vi "Actuators Move Relative Channel.vi"(0 "Notifier Name":string, 2 "Wait to Finish":bool, 5 "Channel":i32, 7 "Step":dbl, 11 "Error In":errorcluster) -> (4 "Notifier Name Out":string, 6 "Channel Out":i32, 15 "Error Out":errorcluster)   [LabVIEW 2025]
uses:
  Actuators Controls/Actuators Note Type.ctl
  Actuators Controls/Actuators Actions.ctl
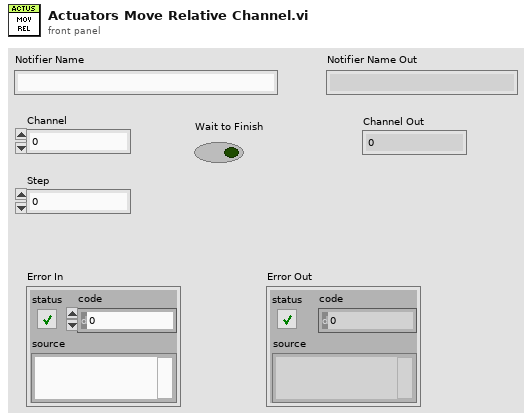
[diagram p1: front panel]
types:
  T1 = typedef "Actuators Note Type.ctl" = cluster{"Actions":T2, "Cmd Received ":bool, "Setpoint":dbl[], "Position":dbl[], "Channel":i32[], "Jog Step":dbl[], "Velocity":dbl[], "Acceleration":dbl[], "Status Bits":u32[], "Moving":bool[]}
  T2 = typedef "Actuators Actions.ctl" = enum16{"Nothing", "Get Position", "Get Acceleration", "Get Velocity", "Get Jog Step", "Set Acceleration", "Set Velocity", "Set Jog Step", "Move Absolute", "Move Relative", "Jog Forward", "Jog Reverse", "Set Moving", "Halt", "Quit"}
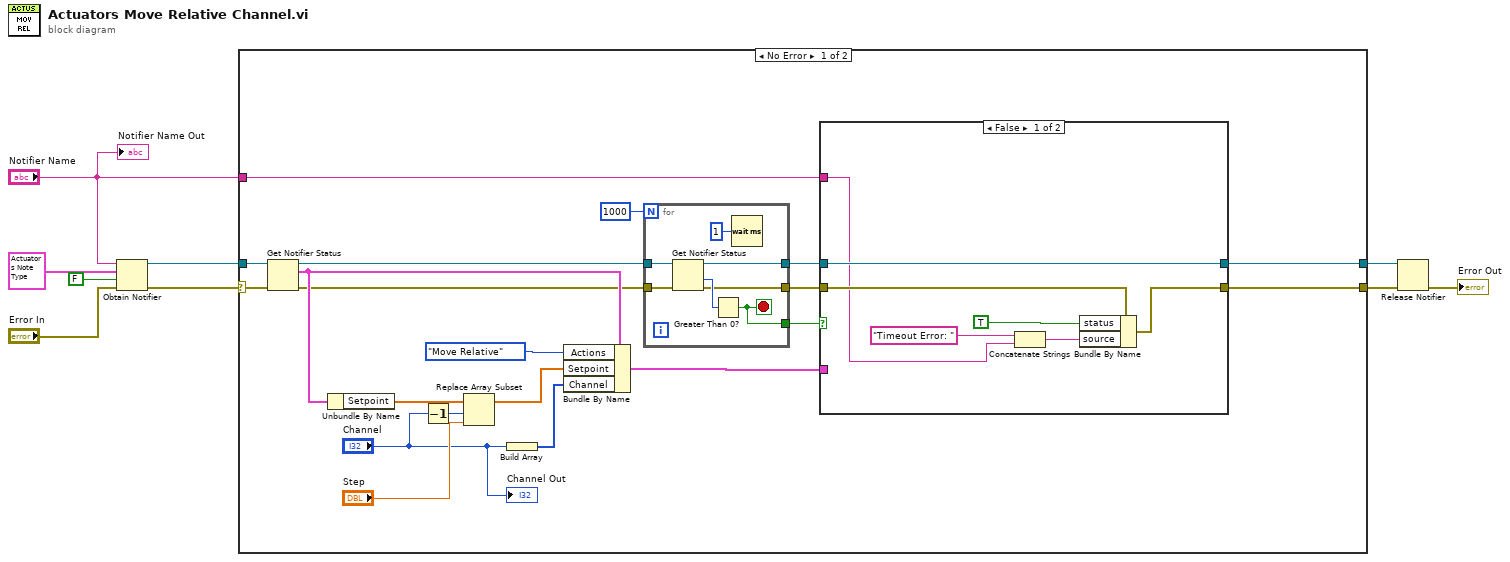
[diagram p0: block diagram]
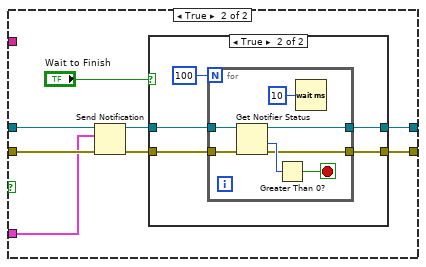
[diagram p2: hidden frame]
diagram:
  n1 = Obtain Notifier(name (unnamed)="Notifier Name", notification data type=T1 {"Actions"=enum."Nothing", "Cmd Received "=FALSE, "Setpoint"=[], "Position"=[], "Channel"=[], "Jog Step"=[], "Velocity"=[], "Acceleration"=[], "Status Bits"=[], "Moving"=[]} ("Actuators Note"), create if not found? (T)=FALSE, error in (no error)="Error In") -> (notifier out=w5:refnum<notifier>, error out=w8:errorcluster)  [unwired: 1 out]
  n2 = case shown="No Error" w8 {
    selector: w8 -> [w23 w66]
    tunnel: w5 -> [w24 w67]
    tunnel: "Notifier Name" -> [w14 _]
    tunnel: [w29 w67] -> w4
    tunnel: [w28 w66] -> w3
    frame No Error {
      n3 = Get Notifier Status(notifier=w24, error in (no error)=w23) -> (notifier out=w20:refnum<notifier>, current notification=w22:T1, error out=w19:errorcluster)  [unwired: 2 out]
      n4 = Unbundle By Name(w22) -> ("Setpoint"=w26:dbl[])
      n5 = Decrement(x="Channel") -> (x-1=w11:i32)
      n6 = Replace Array Subset(array=w26, new element="Step", index=w11) -> (w27:dbl[])
      n7 = Build Array("Channel") -> (w13:i32[])
      n8 = Bundle By Name(cluster=w22, "Actions"=Actuators_Actions."Move Relative", "Setpoint"=w27, "Channel"=w13) -> (w15:T1)
      n9 = for {
        N: 1000 -> [_]
        tunnel: w20 -> [w65]
        tunnel: [w64] -> w18
        tunnel: w19 -> [w61]
        tunnel: [w60] -> w16
        tunnel: [w59] -> w17
        stop <- w60 stop-if-true
        n10 = Get Notifier Status(notifier=w65, error in (no error)=w61) -> (notifier out=w64:refnum<notifier>, # waiting=w63:i32, error out=w59:errorcluster)  [unwired: 2 out]
        n11 = Greater Than 0?(x=w63) -> (x > 0?=w60:bool)
        n12 = Wait (ms)(milliseconds to wait=u32 1) -> ()  [unwired: 1 out]
      }
      n13 = case shown="False" w16 {
        tunnel: [w31 w44] -> w29
        tunnel: [w32 w43] -> w28
        tunnel: w18 -> [w31 w39]
        tunnel: w17 -> [w33 w38]
        tunnel: w15 -> [_ w37]
        tunnel: w14 -> [w30 _]
        frame False {
          n14 = Concatenate Strings("Timeout Error: " ("source"), w30) -> (w36:string)
          n15 = Bundle By Name(cluster=w33, "status"=TRUE, "source"=w36) -> (w32:errorcluster)
        }
        frame True {
          n16 = Send Notification(notification=w37, notifier=w39, error in (no error)=w38) -> (notifier out=w42:refnum<notifier>, error out=w41:errorcluster)
          n17 = case shown="True" "Wait to Finish" {
            tunnel: w42 -> [w46 w50]
            tunnel: w41 -> [w45 w49]
            tunnel: [w45 w48] -> w43
            tunnel: [w46 w47] -> w44
            frame False {
            }
            frame True {
              n18 = for {
                N: 100 -> [_]
                tunnel: w50 -> [w58]
                tunnel: [w57] -> w47
                tunnel: w49 -> [w54]
                tunnel: [w52] -> w48
                stop <- w53 stop-if-true
                n19 = Get Notifier Status(notifier=w58, error in (no error)=w54) -> (notifier out=w57:refnum<notifier>, # waiting=w56:i32, error out=w52:errorcluster)  [unwired: 2 out]
                n20 = Greater Than 0?(x=w56) -> (x > 0?=w53:bool)
                n21 = Wait (ms)(milliseconds to wait=u32 10) -> ()  [unwired: 1 out]
              }
            }
          }
        }
      }
      "Channel Out" <- "Channel"
    }
    frame Error {
    }
  }
  n22 = Release Notifier(notifier=w4, error in (no error)=w3) -> (error out=→"Error Out":errorcluster)  [unwired: 1 in, 2 out]
  "Notifier Name Out" <- "Notifier Name"
